vi "SetDigitalStimTicklish.vi"(8 "error in (no error)":errorcluster, 10 "digital stimuli":T1(array[cluster]), 11 "Serial USB port name":refnum<visa-resource-name>) -> (0 "error in (no error) 2":errorcluster, 3 "Serial USB port name 2":refnum<visa-resource-name>)   [LabVIEW 2015]
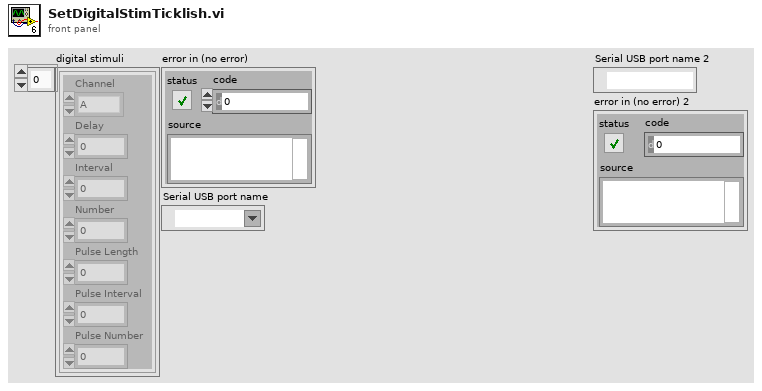
[diagram p1: front panel]
types:
  T1 = cluster{"Channel":enum16{"A", "B", "C", "D", "E", "F", "G", "H", "I", "J", "K", "L", "M", "N", "O", "P", "Q", "R", "S", "T", "U", "V", "W", "X"}, "Delay":dbl, "Interval":dbl, "Number":i32, "Pulse Length":dbl, "Pulse Interval":dbl, "Pulse Number":i32}[]
  T2 = enum16{"A", "B", "C", "D", "E", "F", "G", "H", "I", "J", "K", "L", "M", "N", "O", "P", "Q", "R", "S", "T", "U", "V", "W", "X"}
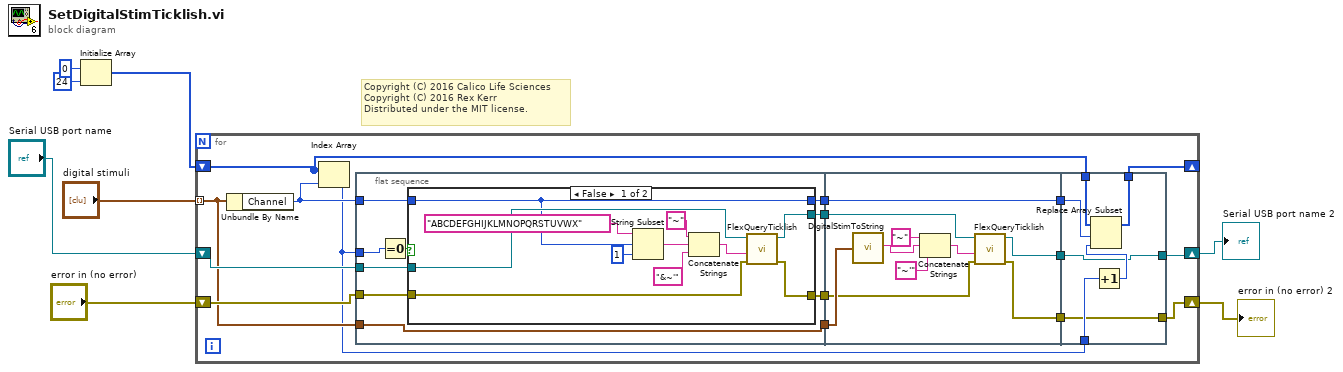
[diagram p0: block diagram]
diagram:
  # "Copyright (C) 2016 Calico Life Sciences\nCopyright (C) 2016 Rex Kerr\nDistributed under the MIT license."
  n1 = Initialize Array(0 ("element"), 24 ("dimension size")) -> (w5:i32[])
  n2 = for {
    tunnel: "digital stimuli" -> [w21] mode=indexing
    shift-right: [w13] -> _
    shift-left: w5 -> [w17]
    shift-right: [w11] -> w2
    shift-left: "Serial USB port name" -> [w23]
    shift-right: [w9] -> w1
    shift-left: "error in (no error)" -> [w24]
    n3 = Unbundle By Name(w21) -> ("Channel"=w22:T2)
    n4 = Index Array(array=w17, index=w22) -> (element=w14:i32)
    n5 = flat-sequence {
      tunnel: w14 -> [w32]
      tunnel: w24 -> [w31]
      tunnel: w23 -> [w30]
      tunnel: w22 -> [w29]
      tunnel: w21 -> [w28]
      tunnel: [w28] -> w20
      tunnel: [w27] -> w19
      tunnel: [w26] -> w18
      tunnel: [w25] -> w15
      tunnel: w20 -> [w55]
      tunnel: w19 -> [w52]
      tunnel: w18 -> [w51]
      tunnel: [w50] -> w16
      tunnel: w15 -> [w50]
      tunnel: [w49] -> w12
      tunnel: [w48] -> w10
      tunnel: w17 -> [w64]
      tunnel: w16 -> [w63]
      tunnel: w14 -> [w62]
      tunnel: [w60] -> w13
      tunnel: w12 -> [w59]
      tunnel: [w59] -> w11
      tunnel: w10 -> [w58]
      tunnel: [w58] -> w9
      frame #0 {
        n6 = Equal To 0?(x=w32) -> (x = 0?=w33:bool)
        n7 = case shown="False" w33 {
          tunnel: w31 -> [w40 w46]
          tunnel: w30 -> [w39 w47]
          tunnel: w29 -> [w34 w45]
          tunnel: [w36 w47] -> w27
          tunnel: [w35 w46] -> w26
          tunnel: [w34 w45] -> w25
          frame False {
            n8 = String Subset(string="ABCDEFGHIJKLMNOPQRSTUVWX", offset (0)=w34, length (rest)=1 ("length (rest)")) -> (substring=w44:string)
            n9 = Concatenate Strings("~" ("string"), w44, "&~'" ("string")) -> (w41:string)
            n10 = call "FlexQueryTicklish.vi"("error in (no error)"=w40, "write buffer"=w41, "Serial USB port name"=w39) -> ("error out"=w35:errorcluster, "Serial USB port name out"=w36:refnum<visa-resource-name>)  [unwired: 6 in, 1 out]
          }
          frame True {
          }
        }
      }
      frame #1 {
        n11 = call "DigitalStimToString.vi"("digital stimulus"=w55) -> ("stimulus set string"=w56:string)  [unwired: 4 in]
        n12 = Concatenate Strings("~" ("string"), w56, "~'" ("string")) -> (w53:string)
        n13 = call "FlexQueryTicklish.vi"("error in (no error)"=w51, "write buffer"=w53, "Serial USB port name"=w52) -> ("error out"=w48:errorcluster, "Serial USB port name out"=w49:refnum<visa-resource-name>)  [unwired: 6 in, 1 out]
      }
      frame #2 {
        n14 = Increment(x=w62) -> (x+1=w61:i32)
        n15 = Replace Array Subset(array=w64, new element=w61, index=w63) -> (w60:i32[])
      }
    }
  }
  "Serial USB port name 2" <- w2
  "error in (no error) 2" <- w1
